vi "Reset Iterations.vi"(8 "error in (no error)":errorcluster, 11 "Function in":refnum<class "Function.lvclass">) -> (0 "error out":errorcluster, 3 "Function out":refnum<class "Function.lvclass">)   [LabVIEW 2016]
uses:
  <userlib>/Common Components/Function Actor/Function.lvclass
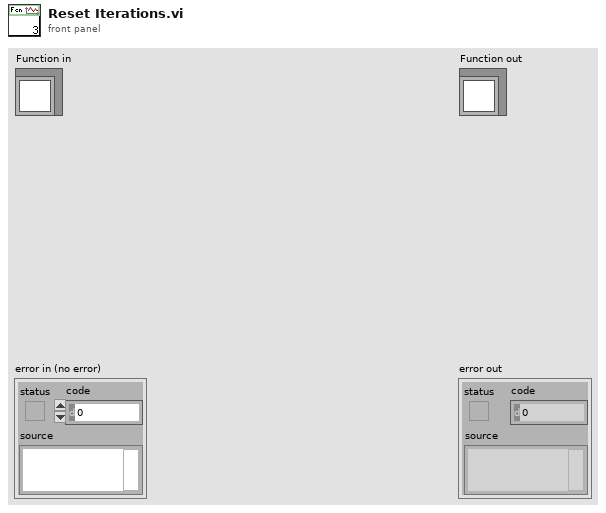
[diagram p1: front panel]
types:
  T1 = typedef "Iteration Count.ctl" = cluster{"Desired Iterations":i32, "Current":i32}
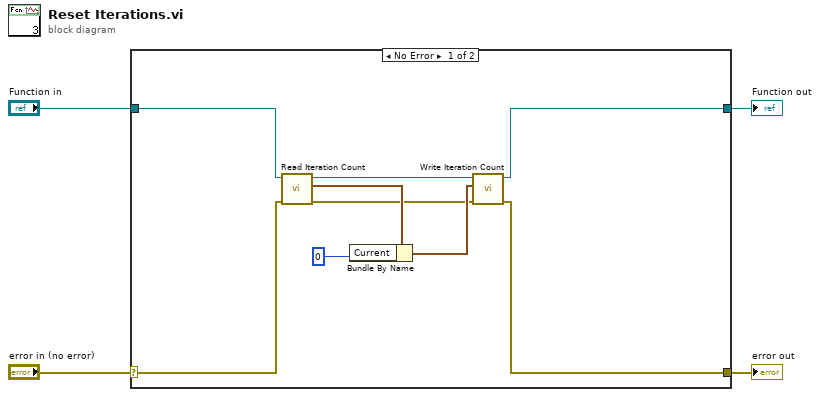
[diagram p0: block diagram]
diagram:
  n1 = case shown="No Error" "error in (no error)" {
    selector: "error in (no error)" -> [w6 w15]
    tunnel: [w5 w15] -> w3
    tunnel: [w8 w14] -> w1
    tunnel: "Function in" -> [w9 w14]
    frame No Error {
      n2 = call <userlib>:"Read Iteration Count.vi"("error in (no error)"=w6, "Function in"=w9) -> ("error out"=w7:errorcluster, "Iteration Count"=w13:T1, "Function out"=w10:refnum<class "Function.lvclass">)  [unwired: 7 in]
      n3 = Bundle By Name(cluster=w13, "Current"=0) -> (w11:T1)
      n4 = call <userlib>:"Write Iteration Count.vi"("error in (no error)"=w7, "Iteration Count"=w11, "Function in"=w10) -> ("error out"=w5:errorcluster, "Function out"=w8:refnum<class "Function.lvclass">)  [unwired: 7 in]
    }
    frame Error {
    }
  }
  "error out" <- w3
  "Function out" <- w1
